vi "key_empty.vi"(10 "Key (search)":T1, 11 "Key (node)":T1) -> (2 "Equal?":bool, 3 "Empty?":bool)   [LabVIEW 2015, in "binary_tree.lvlib"]
uses:
  binary_tree.lvlib
  _Controls/node_key.ctl
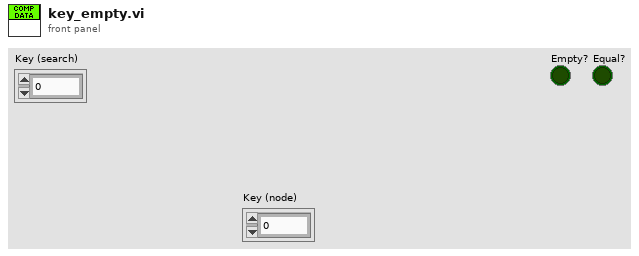
[diagram p1: front panel]
types:
  T1 = typedef "binary_tree.lvlib/node_key.ctl" = cluster{dbl}
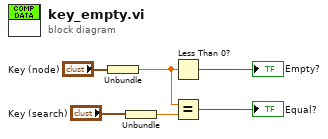
[diagram p0: block diagram]
diagram:
  n1 = Unbundle("Key (node)") -> (w2:dbl)
  n2 = Unbundle("Key (search)") -> (w3:dbl)
  n3 = Less Than 0?(x=w2) -> (x < 0?=→"Empty?":bool)
  n4 = Equal?(x=w2, y=w3) -> (x = y?=→"Equal?":bool)
